vi "전략1 2차업그레이드.vi"() -> ()   [LabVIEW 2015]
uses:
  <vilib>/NXT/Block Support/NXT_InputPort.ctl
  <vilib>/NXT/Subs/MotorOutput.ctl
  <vilib>/NXT/Dual Mode Library/Sensors/Sonar_cm.vi
  <vilib>/NXT/Dual Mode Library/Motors/MotorOn.vi
  <vilib>/NXT/Dual Mode Library/Waits/Wait_Rotation.vi
  <vilib>/NXT/Dual Mode Library/Waits/Wait_Num.vi
  <vilib>/NXT/Dual Mode Library/Sensors/Light_On.vi
  <vilib>/NXT/Dual Mode Library/Motors/MotorReverse.vi
panel:
  in  "정지":bool
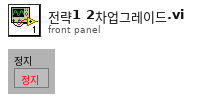
[diagram p1: front panel]
types:
  T1 = typedef "MotorOutput.ctl" = u8
  T2 = typedef "NXT_InputPort.ctl" = u32
  T3 = typedef "LVHSConnector.ctl" = refnum<class "BrickReference.lvclass">
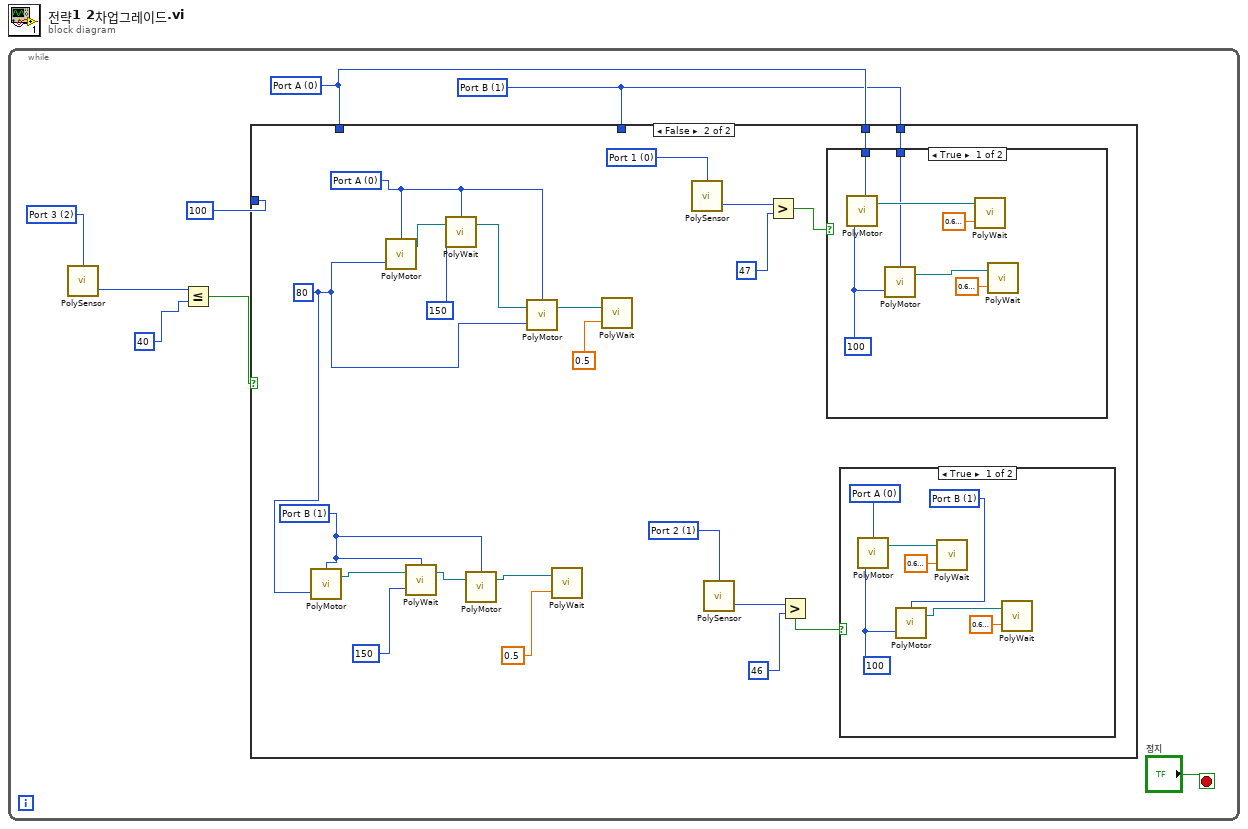
[diagram p0: block diagram]
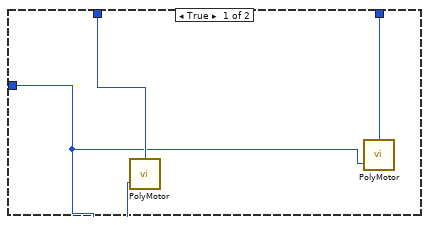
[diagram p2: hidden frame]
diagram:
  n1 = while {
    stop <- "정지" stop-if-true
    w1 = T1 1 items=["Port A", "Port B", "Port C", "All Ports"] ("Output Port (All Ports)")
    w2 = T1 0 items=["Port A", "Port B", "Port C", "All Ports"] ("Output Port (All Ports)")
    w5 = T2 2 items=["Port 1", "Port 2", "Port 3", "Port 4"] ("Input Port")
    n2 = call-poly <vilib>:"PolySensor.vi"("Port (Port 4)"=w5) -> ("Distance (cm)"=w3:i16)  [unwired: 2 in, 1 out]
    n3 = Less Or Equal?(x=w3, y=40) -> (x <= y?=w6:bool)
    n4 = case shown="False" w6 {
      tunnel: w2 -> [w11 _]
      tunnel: 100 ("Power (75)") -> [w9 _]
      tunnel: w1 -> [w10 _]
      tunnel: w2 -> [_ w20]
      tunnel: w1 -> [_ w19]
      frame True {
        n5 = call-poly <vilib>:"PolyMotor.vi"("Power (75)"=w9, "Output Port (All Ports)"=w11) -> ()  [unwired: 2 in, 1 out]
        n6 = call-poly <vilib>:"PolyMotor.vi"("Power (75)"=w9, "Output Port (All Ports)"=w10) -> ()  [unwired: 2 in, 1 out]
      }
      frame False {
        w12 = T1 1 items=["Port A", "Port B", "Port C", "All Ports"] ("Output Port (All Ports)")
        w22 = T2 1 items=["Port 1", "Port 2", "Port 3", "Port 4"] ("Input Port")
        w21 = T2 0 items=["Port 1", "Port 2", "Port 3", "Port 4"] ("Input Port")
        w15 = 80 ("Power (75)")
        w29 = T1 0 items=["Port A", "Port B", "Port C", "All Ports"] ("Output Port (All Ports)")
        n7 = call-poly <vilib>:"PolyMotor.vi"("Power (75)"=w15, "Output Port (All Ports)"=w12) -> ("NXT/EV3"=w16:T3)  [unwired: 2 in]
        n8 = call-poly <vilib>:"PolyMotor.vi"("Power (75)"=w15, "Output Port (All Ports)"=w29) -> ("NXT/EV3"=w34:T3)  [unwired: 2 in]
        n9 = call-poly <vilib>:"PolyWait.vi"("Position Change (180)"=150, "NXT/EV3"=w16, "Port (Port A)"=w12) -> ("NXT/EV3"=w17:T3)  [unwired: 1 in]
        n10 = call-poly <vilib>:"PolyWait.vi"("Position Change (180)"=150, "NXT/EV3"=w34, "Port (Port A)"=w29) -> ("NXT/EV3"=w32:T3)  [unwired: 1 in]
        n11 = call-poly <vilib>:"PolyMotor.vi"("NXT/EV3"=w17, "Output Port (All Ports)"=w12) -> ("NXT/EV3"=w18:T3)  [unwired: 2 in]
        n12 = call-poly <vilib>:"PolyMotor.vi"("Power (75)"=w15, "NXT/EV3"=w32, "Output Port (All Ports)"=w29) -> ("NXT/EV3"=w31:T3)  [unwired: 1 in]
        n13 = call-poly <vilib>:"PolyWait.vi"("Time (1 sec)"=sgl 0.5, "NXT/EV3"=w18) -> ()  [unwired: 2 in, 1 out]
        n14 = call-poly <vilib>:"PolyWait.vi"("Time (1 sec)"=sgl 0.5, "NXT/EV3"=w31) -> ()  [unwired: 2 in, 1 out]
        n15 = call-poly <vilib>:"PolySensor.vi"("Port (Port 3)"=w21) -> ("Scaled Value"=w25:i16)  [unwired: 2 in, 1 out]
        n16 = call-poly <vilib>:"PolySensor.vi"("Port (Port 3)"=w22) -> ("Scaled Value"=w28:i16)  [unwired: 2 in, 1 out]
        n17 = Greater?(x=w25, y=47) -> (0:w23:bool)
        n18 = Greater?(x=w28, y=46) -> (0:w26:bool)
        n19 = case shown="True" w23 {
          tunnel: w20 -> [w39 _]
          tunnel: w19 -> [w36 _]
          frame True {
            w35 = 100 ("Power (75)")
            n20 = call-poly <vilib>:"PolyMotor.vi"("Power (75)"=w35, "Output Port (All Ports)"=w39) -> ("NXT/EV3"=w41:T3)  [unwired: 2 in]
            n21 = call-poly <vilib>:"PolyMotor.vi"("Power (75)"=w35, "Output Port (All Ports)"=w36) -> ("NXT/EV3"=w37:T3)  [unwired: 2 in]
            n22 = call-poly <vilib>:"PolyWait.vi"("Time (1 sec)"=sgl 0.7 ("Time (sec)"), "NXT/EV3"=w41) -> ()  [unwired: 2 in, 1 out]
            n23 = call-poly <vilib>:"PolyWait.vi"("Time (1 sec)"=sgl 0.7 ("Time (sec)"), "NXT/EV3"=w37) -> ()  [unwired: 2 in, 1 out]
          }
          frame False {
          }
        }
        n24 = case shown="True" w26 {
          frame True {
            w43 = T1 1 items=["Port A", "Port B", "Port C", "All Ports"] ("Output Port (All Ports)")
            w46 = T1 0 items=["Port A", "Port B", "Port C", "All Ports"] ("Output Port (All Ports)")
            w42 = 100 ("Power (75)")
            n25 = call-poly <vilib>:"PolyMotor.vi"("Power (75)"=w42, "Output Port (All Ports)"=w46) -> ("NXT/EV3"=w48:T3)  [unwired: 2 in]
            n26 = call-poly <vilib>:"PolyMotor.vi"("Power (75)"=w42, "Output Port (All Ports)"=w43) -> ("NXT/EV3"=w44:T3)  [unwired: 2 in]
            n27 = call-poly <vilib>:"PolyWait.vi"("Time (1 sec)"=sgl 0.7 ("Time (sec)"), "NXT/EV3"=w48) -> ()  [unwired: 2 in, 1 out]
            n28 = call-poly <vilib>:"PolyWait.vi"("Time (1 sec)"=sgl 0.7 ("Time (sec)"), "NXT/EV3"=w44) -> ()  [unwired: 2 in, 1 out]
          }
          frame False {
          }
        }
      }
    }
  }
